vi "ROI grp-Window-Edit POI group name.vi"() -> (1 "Group Name out":string, 3 "Cancelled":bool)   [LabVIEW 2020]
uses:
  Typedefs/Get-Set-Clear Control.ctl
  Globals/gl_ROI grp window globals.vi
  Global Variables/General Globals.vi
panel:
  in  "Cancel":bool
  in  "OK":bool
  in  "Group name ctrl":string caption="Enter a new name for the selected group"
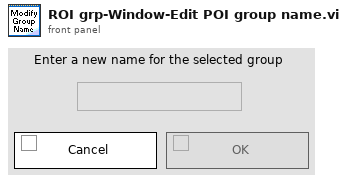
[diagram p1: front panel]
types:
  T1 = typedef "Get-Set-Clear Control.ctl" = enum16{"Get", "Set", "Clear"}
  T2 = typedef "ROI grp-window ctrl refs.ctl" = cluster{"This VI":refnum<vi>, "Pane":refnum<vi>, "Table":refnum<vi>}
  T3 = typedef "ROI group info cluster.ctl" = cluster{"Group name":string, "# ROI in group":i32, "ROI numbers in group":i32[], "Group region specifier cluster":T4}
  T4 = typedef "ROI Descriptor" = cluster{"Global Rectangle":i32[], "Contours":cluster{"ID":enum32{"External", "Internal"}, "Type":u32, "Coordinates":i32[]}[]}
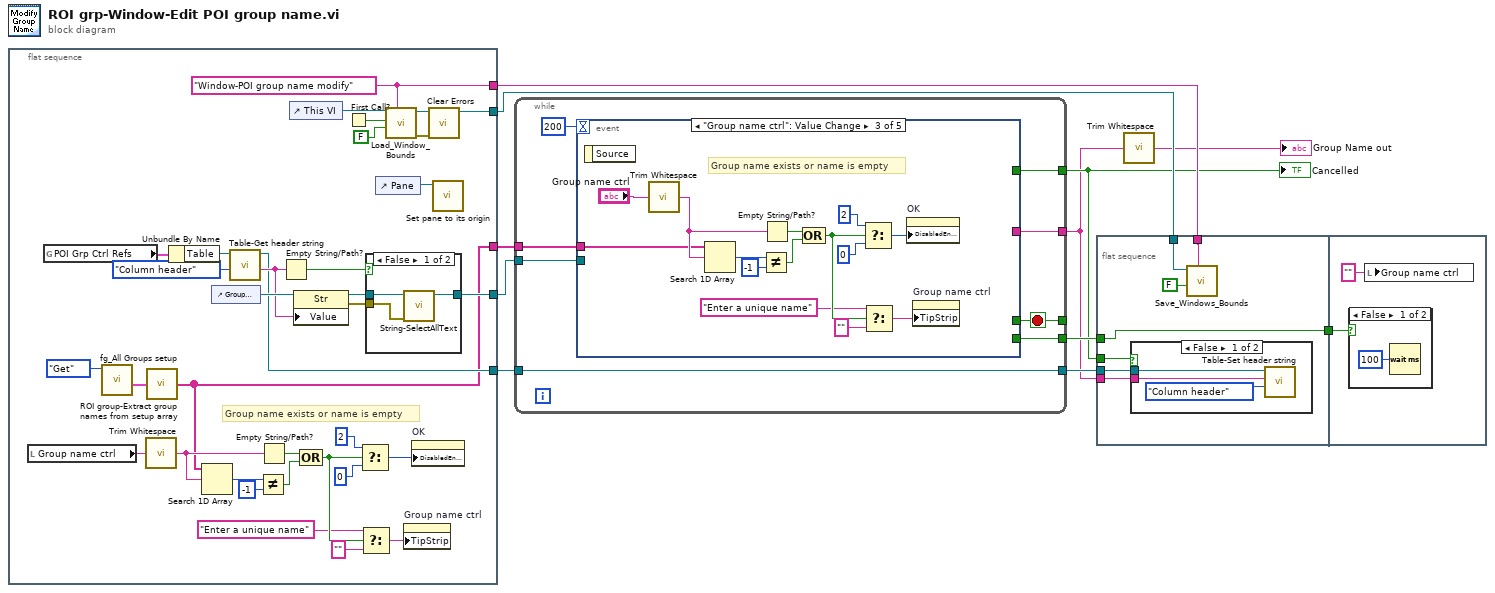
[diagram p0: block diagram]
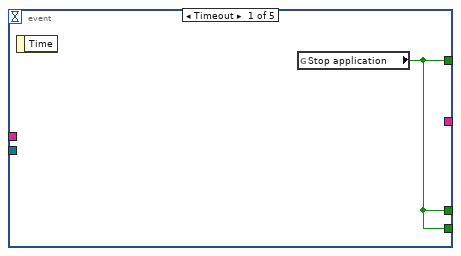
[diagram p5: hidden frame]
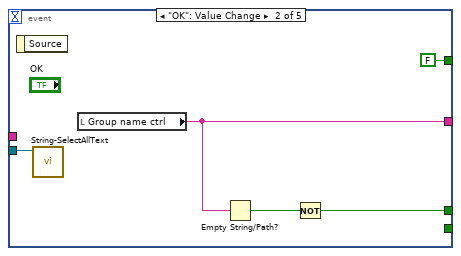
[diagram p6: hidden frame]
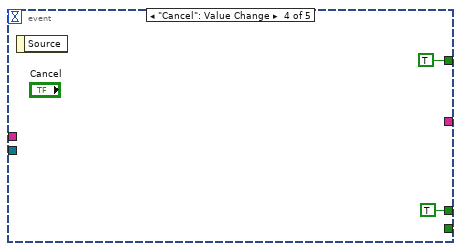
[diagram p7: hidden frame]
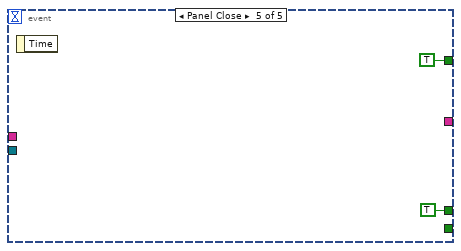
[diagram p8: hidden frame]
diagram:
  n1 = flat-sequence {
    tunnel: [w40] -> w9
    tunnel: [w39] -> w7
    tunnel: [w31] -> w8
    tunnel: [w30] -> w5
    tunnel: [w13] -> w1
    frame #0 {
      w40 = "Window-POI group name modify" ("Window Name (i.e. Key)")
      # "Group name exists or name is empty"
      n2 = local read "Group name ctrl"() -> (w14:string)
      n3 = global read "gl_ROI grp window globals.vi" "POI Grp Ctrl Refs"() -> (w29:T2)
      n4 = call "fg_All Groups setup.vi"("Function"=Get-Set-Clear_Control."Get") -> ("Groups setup out"=w16:T3[])  [unwired: 9 in, 1 out]
      n5 = call <vilib>:"Trim Whitespace.vi"("string"=w14) -> ("trimmed string"=w20:string)  [unwired: 1 in]
      n6 = call "ROI group-Extract group names from setup array.vi"("Groups setup"=w16) -> ("Group Names Array"=w13:string[])
      n7 = Unbundle By Name(w29) -> ("Table"=w38:refnum<vi>)
      n8 = Search 1D Array(1D array=w13, element=w20) -> (index of element=w26:i32)  [unwired: 1 in]
      n9 = control-ref of="Group name ctrl"() -> (w36:refnum<vi>)
      n10 = call <userlib>:"Table-Get header string.vi"("Row/Column"=enum16{"Row header", "Column header"}."Column header", "Table"=w38) -> ("Column header"=w33:string, "Table out"=w30:refnum<vi>)  [unwired: 7 in, 1 out]
      n11 = Not Equal?(x=w26, y=-1) -> (x != y?=w23:bool)
      n12 = Empty String/Path?(string/path=w20) -> (empty?=w24:bool)
      n13 = Empty String/Path?(string/path=w33) -> (empty?=w32:bool)
      n14 = control-ref of="This VI"() -> (w28:refnum<vi>)
      n15 = property on="Property Node" class="Str"(reference=w36, "Value"=w33) -> (reference out=w35:refnum<vi>, error out=w34:errorcluster)  [unwired: 1 in]
      n16 = Compound Arithmetic op=OR(w24, w23) -> (w19:bool)
      n17 = First Call?() -> (First Call?: T/F=w42:bool)
      n18 = Select(t=2, s=w19, f=0) -> (s? t:f=w12:i32)
      n19 = Select(t="Enter a unique name" ("Tip Strip"), s=w19, f="") -> (s? t:f=w27:string)
      n20 = case shown="False" w32 {
        tunnel: w35 -> [w47 w48]
        tunnel: w34 -> [w46 _]
        tunnel: [w45 w48] -> w31
        frame False {
          n21 = call <userlib>:"String-SelectAllText.vi"("error in (no error)"=w46, "String control ref"=w47) -> ("reference out"=w45:refnum<vi>)  [unwired: 8 in, 1 out]
        }
        frame True {
        }
      }
      n22 = control-ref of="Pane"() -> (w44:refnum<vi>)
      n23 = call "Load_Window_Bounds.vi"("Window Name (i.e. Key)"=w40, "Disable"=FALSE, "First Call"=w42, "Window VI's Ref"=w28) -> ("error out"=w41:errorcluster, "reference out"=w39:refnum<vi>)  [unwired: 4 in, 2 out]
      n24 = property on="Group name ctrl" class="Str"("TipStrip"=w27) -> ()  [unwired: 2 in, 2 out]
      n25 = property on="OK" class="Bool"("DisabledEnum"=w12) -> ()  [unwired: 2 in, 2 out]
      n26 = call <vilib>:"Clear Errors.vi"("error in (no error)"=w41) -> ()  [unwired: 5 in, 2 out]
      n27 = call <userlib>:"Set pane to its origin.vi"("Pane Reference"=w44) -> ()  [unwired: 9 in, 2 out]
    }
  }
  n28 = while {
    tunnel: [w56] -> _
    tunnel: [w54] -> w4
    tunnel: [w53] -> w11
    tunnel: [w52] -> w2
    tunnel: w8 -> [w51]
    tunnel: [w50] -> w6
    tunnel: w5 -> [w50]
    tunnel: w1 -> [w49]
    stop <- w56 stop-if-true
    n29 = event shown="[2] \"Group name ctrl\": Value Change" {
      selector: _ -> [_ _ _ _ _]
      dyn-events: _ -> [_ _ _ _ _]
      timeout: 200 -> [_ _ _ _ _]
      tunnel: [w57 w60 _ TRUE TRUE] -> w56
      tunnel: [w57 FALSE ("Cancel") _ TRUE ("Cancel") TRUE ("Cancel")] -> w54
      tunnel: [w57 _ _ _ _] -> w53
      tunnel: [_ w58 _ _ _] -> w52
      tunnel: w51 -> [_ w59 _ _ _]
      tunnel: w49 -> [_ _ w65 _ _]
      event Timeout {
        n30 = event-data() -> ()  [unwired: 1 in, 1 out]
        n31 = global read "General Globals.vi" "Stop application"() -> (w57:bool)
      }
      event "OK": Value Change {
        n32 = event-data() -> ()  [unwired: 1 in, 1 out]
        n33 = call <userlib>:"String-SelectAllText.vi"("String control ref"=w59) -> ()  [unwired: 9 in, 2 out]
        n34 = local read "Group name ctrl"() -> (w58:string)
        n35 = Empty String/Path?(string/path=w58) -> (empty?=w61:bool)
        n36 = Not(x=w61) -> (.not. x?=w60:bool)
      }
      event "Group name ctrl": Value Change {
        # "Group name exists or name is empty"
        n37 = event-data() -> ()  [unwired: 1 in, 1 out]
        n38 = call <vilib>:"Trim Whitespace.vi"("string"="Group name ctrl") -> ("trimmed string"=w70:string)  [unwired: 1 in]
        n39 = Search 1D Array(1D array=w65, element=w70) -> (index of element=w76:i32)  [unwired: 1 in]
        n40 = Not Equal?(x=w76, y=-1) -> (x != y?=w73:bool)
        n41 = Empty String/Path?(string/path=w70) -> (empty?=w74:bool)
        n42 = Compound Arithmetic op=OR(w74, w73) -> (w69:bool)
        n43 = Select(t=2, s=w69, f=0) -> (s? t:f=w63:i32)
        n44 = Select(t="Enter a unique name" ("Tip Strip"), s=w69, f="") -> (s? t:f=w68:string)
        n45 = property on="OK" class="Bool"("DisabledEnum"=w63) -> ()  [unwired: 2 in, 2 out]
        n46 = property on="Group name ctrl" class="Str"("TipStrip"=w68) -> ()  [unwired: 2 in, 2 out]
      }
      event "Cancel": Value Change {
        n47 = event-data() -> ()  [unwired: 1 in, 1 out]
      }
      event Panel Close {
        n48 = event-data() -> ()  [unwired: 1 in, 1 out]
      }
    }
  }
  "Cancelled" <- w4
  n49 = flat-sequence {
    tunnel: [w87] -> w10
    tunnel: w9 -> [w82]
    tunnel: w11 -> [w87]
    tunnel: w7 -> [w83]
    tunnel: w6 -> [w86]
    tunnel: w2 -> [w85]
    tunnel: w4 -> [w84]
    tunnel: w10 -> [w92]
    frame #0 {
      n50 = case shown="False" w84 {
        tunnel: w86 -> [w90 _]
        tunnel: w85 -> [w88 _]
        frame False {
          n51 = call <userlib>:"Table-Set header string.vi"("Row/Column"=enum16{"Row header", "Column header"}."Column header", "Column header string"=w88, "Table"=w90) -> ()  [unwired: 7 in, 2 out]
        }
        frame True {
        }
      }
      n52 = call "Save_Windows_Bounds.vi"("Window Name (i.e. Key)"=w82, "Front Panel Window:Open"=FALSE, "Window VI's Ref"=w83) -> ()  [unwired: 8 in, 1 out]
    }
    frame #1 {
      n53 = case shown="False" w92 {
        frame False {
          n54 = Wait (ms)(milliseconds to wait=u32 100) -> ()  [unwired: 1 out]
        }
        frame True {
        }
      }
      n55 = local write "Group name ctrl"("" ("Group name ctrl")) -> ()
    }
  }
  n56 = call <vilib>:"Trim Whitespace.vi"("string"=w2) -> ("trimmed string"=→"Group Name out":string)  [unwired: 1 in]
